vi "Constructor.vi"(5 "TimeZoneInfoId":string, 6 "MeasureExecutionStatus":T1=enum."NOT_COMPLETED", 7 "MeasureTime":timestamp, 8 "error in":errorcluster, 10 "Value":timestamp, 11 "Name":string) -> (0 "error out":errorcluster, 3 "DateTimeMeasure":refnum<class "DateTimeMeasure.lvclass">)   [LabVIEW 2021, in "ProligentXMLGenerator.lvlib" / "DateTimeMeasure.lvclass"]
uses:
  DateTimeMeasure.lvclass
  DateTimeMeasure.lvclass/DateTimeMeasure.ctl
  Measure/Measure.lvclass
  Base/MeasureKind/Value.ctl
  Base/MeasureKind/MeasureKind.lvclass
  Base/DateTime/DateTime.lvclass
  Data.ctl
  C:/Projects/proligent-xml-generator-labview/src/ProligentXMLGenerator/Measure/Measure/Measure.lvclass
  C:/Projects/proligent-xml-generator-labview/src/ProligentXMLGenerator/Measure/DateTimeMeasure/DateTimeMeasure.lvclass
  Base/ExecutionStatus/Value.ctl
  Base/ExecutionStatus/ExecutionStatus.lvclass
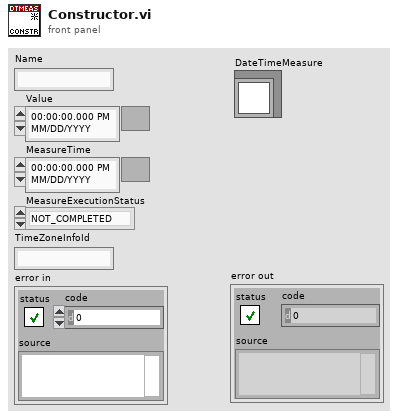
[diagram p1: front panel]
types:
  T1 = typedef "ProligentXMLGenerator.lvlib/ExecutionStatus.lvclass/Value.ctl" = enum16{"PASS", "FAIL", "NOT_COMPLETED", "ABORTED"}
  T2 = typedef "ProligentXMLGenerator.lvlib/DateTimeMeasure.lvclass/Data.ctl" = cluster{"Value":refnum<class "DateTime.lvclass">, "TimeZoneInfoId":string}
  T3 = typedef "ProligentXMLGenerator.lvlib/MeasureKind.lvclass/Value.ctl" = enum16{"REAL", "BOOL", "INTEGER", "STRING", "DATETIME"}
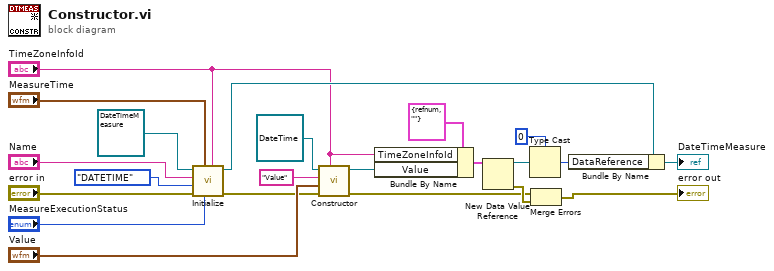
[diagram p0: block diagram]
diagram:
  n1 = call "Initialize.vi"("TimeZoneInfoId"="TimeZoneInfoId", "MeasureExecutionStatus"="MeasureExecutionStatus", "MeasureTime"="MeasureTime", "error in"="error in", "Type"=Value."DATETIME", "Name"="Name", "Measure in"=refnum<class "DateTimeMeasure.lvclass"> refnum ("ProligentResultProcessor:DateTimeMeasure")) -> ("error out"=w8:errorcluster, "Measure out"=w17:refnum<class "DateTimeMeasure.lvclass">)  [unwired: 3 in]
  n2 = call-dynamic "Constructor.vi"("TimeZoneInfoId"="TimeZoneInfoId", "error in"=w8, "Value"="Value", "Name"="Value", "DateTime in"=refnum<class "DateTime.lvclass"> refnum ("ProligentResultProcessor:DateTime")) -> ("error out"=w7:errorcluster, "DateTime out"=w5:refnum<class "DateTime.lvclass">)  [unwired: 5 in]
  n3 = Bundle By Name(cluster=T2 {"Value"=refnum, "TimeZoneInfoId"=""} ("Data"), "TimeZoneInfoId"="TimeZoneInfoId", "Value"=w5) -> (w6:T2)
  n4 = New Data Value Reference(data value=w6) -> (data value reference=w18:refnum<data-value>, error out=w21:errorcluster)  [unwired: 1 in]
  n5 = Type Cast(type=u64 0, x=w18) -> (*(type *) &x=w20:u64)
  n6 = Merge Errors(w7, w21) -> (→"error out":errorcluster)
  n7 = Bundle By Name(cluster=w17, "DataReference"=w20) -> (→"DateTimeMeasure":refnum<class "DateTimeMeasure.lvclass">)
